vi "RSZVB Get Marker Search Mode.vi"(8 "error in (no error)":errorcluster {"code" format="%.0x"}, 9 "Marker (1)":i32=1, 10 "Channel (Trace) (1)":i32=1, 11 "VISA session":refnum<visa-resource-name>) -> (0 "error out":errorcluster {"code" format="%.0x"}, 1 "Search Mode":i32, 3 "dup VISA session":refnum<visa-resource-name>)   [LabVIEW 2011]
doc: "This VI returns the bandfilter search mode.\n\nRemote-control command(s):\nCALCulate<Chn>:MARKer<Mk>:FUNCtion:BWIDth:MODE?"
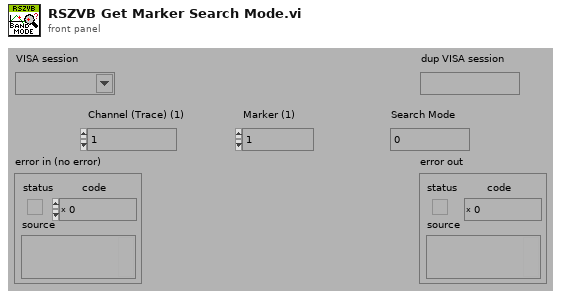
[diagram p1: front panel]
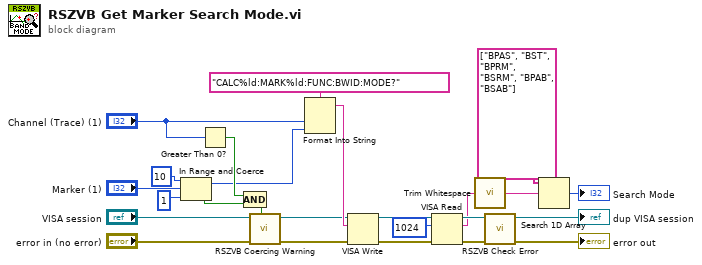
[diagram p0: block diagram]
diagram:
  n1 = In Range and Coerce(upper limit=10, x="Marker (1)", lower limit=1) -> (coerced(x)=w4:i32, In Range?=w25:bool)
  n2 = Greater Than 0?(x="Channel (Trace) (1)") -> (x > 0?=w24:bool)
  n3 = Compound Arithmetic op=AND(w24, w25) -> (w22:bool)
  n4 = call "RSZVB Coercing Warning.vi"("In Range?"=w22, "error in (no error)"="error in (no error)", "VISA session"="VISA session") -> ("error out"=w18:errorcluster, "dup VISA session"=w17:refnum<visa-resource-name>)  [unwired: 7 in]
  n5 = Format Into String(format string="CALC%ld:MARK%ld:FUNC:BWID:MODE?", "Channel (Trace) (1)", w4) -> (resulting string=w23:string)  [unwired: 2 in, 1 out]
  n6 = VISA Write(VISA resource name=w17, write buffer=w23, error in (no error)=w18) -> (VISA resource name out=w10:refnum<visa-resource-name>, error out=w9:errorcluster)  [unwired: 1 out]
  n7 = VISA Read(VISA resource name=w10, byte count=u32 1024 ("byte count (0)"), error in (no error)=w9) -> (VISA resource name out=w12:refnum<visa-resource-name>, read buffer=w2:string, error out=w11:errorcluster)  [unwired: 1 out]
  n8 = call <vilib>:"Trim Whitespace.vi"("string"=w2) -> ("trimmed string"=w6:string)  [unwired: 1 in]
  n9 = call "RSZVB Check Error.vi"("error in (no error)"=w11, "VISA session"=w12) -> ("error out"=→"error out":errorcluster, "dup VISA session"=→"dup VISA session":refnum<visa-resource-name>)  [unwired: 8 in]
  n10 = Search 1D Array(1D array=string[] ["BPAS", "BST", "BPRM", "BSRM", "BPAB", "BSAB"], element=w6) -> (index of element=→"Search Mode":i32)  [unwired: 1 in]
